vi "RestartIfDisconnected.vi"(8 "error in (no error)":errorcluster, 9 "connection timeout":i32=-1, 11 "NetworkStreamWriter in":refnum<class "NetworkStreamWriter.lvclass">) -> (0 "error out":errorcluster, 3 "NetworkStreamWriter out":refnum<class "NetworkStreamWriter.lvclass">)   [LabVIEW 2011, in "NetworkStreamWriter.lvclass"]
uses:
  NetworkStreamWriter.lvclass
  NetworkStreamWriter.lvclass/NetworkStreamWriter.ctl
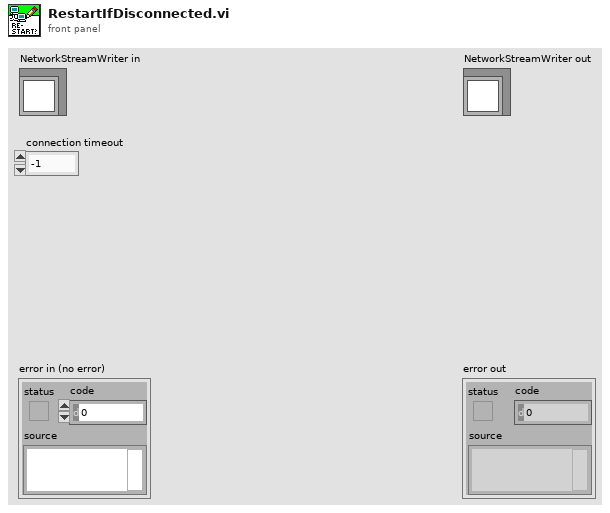
[diagram p1: front panel]
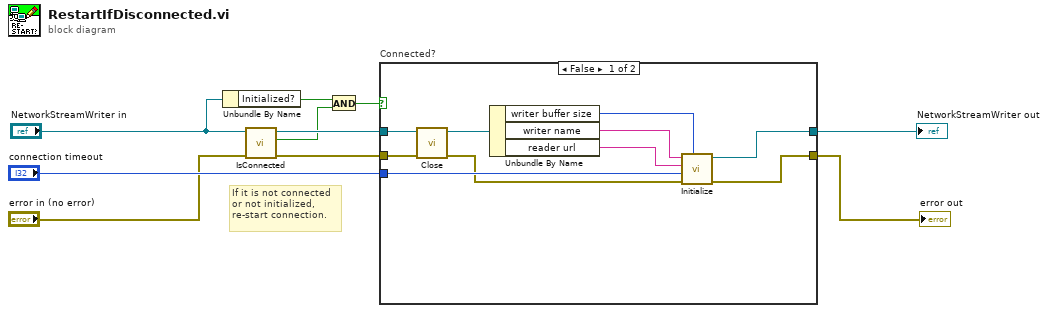
[diagram p0: block diagram]
diagram:
  # "If it is not connected\nor not initialized,\nre-start connection."
  n1 = Unbundle By Name("NetworkStreamWriter in") -> ("Initialized?"=w2:bool)
  n2 = call "IsConnected.vi"("error in (no error)"="error in (no error)", "NetworkStreamWriter in"="NetworkStreamWriter in") -> ("error out"=w4:errorcluster, "Connected?"=w1:bool, "NetworkStreamWriter out"=w5:refnum<class "NetworkStreamWriter.lvclass">)  [unwired: 7 in]
  n3 = And(x=w2, y=w1) -> (x .and. y?=w3:bool)
  n4 = case "Connected?" shown="False" w3 {
    tunnel: w5 -> [w18 w22]
    tunnel: w4 -> [w17 w21]
    tunnel: [w12 w22] -> w9
    tunnel: [w11 w21] -> w6
    tunnel: "connection timeout" -> [w20 _]
    frame False {
      n5 = call "Close.vi"("error in (no error)"=w17, "NetworkStreamWriter in"=w18) -> ("error out"=w13:errorcluster, "NetworkStreamWriter out"=w16:refnum<class "NetworkStreamWriter.lvclass">)  [unwired: 8 in]
      n6 = Unbundle By Name(w16) -> ("writer buffer size"=w19:i32, "writer name"=w15:string, "reader url"=w14:string)
      n7 = call "Initialize.vi"("writer buffer size"=w19, "error in (no error)"=w13, "connection timeout"=w20, "reader url"=w14, "writer name"=w15) -> ("error out"=w11:errorcluster, "NetworkStreamWriter out"=w12:refnum<class "NetworkStreamWriter.lvclass">)  [unwired: 4 in, 1 out]
    }
    frame True {
    }
  }
  "error out" <- w6
  "NetworkStreamWriter out" <- w9
